vi "Append.vi"(8 "error in":errorcluster, 10 "Digital Waveform in":digitalwaveform(waveform)={"t0"=timestamp(0 s since 1904-01-01), "dt"=1.0, "Y"={"transitions"=[], "data"=[]}}, 11 "Digital Waveform Chart in":refnum<class "Digital Waveform Chart.lvclass">) -> (0 "error out":errorcluster, 2 "Digital Waveform out":digitalwaveform(waveform)={"t0"=timestamp(0 s since 1904-01-01), "dt"=1.0, "Y"={"transitions"=[], "data"=[]}}, 3 "Digital Waveform Chart out":refnum<class "Digital Waveform Chart.lvclass">)   [LabVIEW 2024, in "Digital Waveform Chart.lvclass"]
uses:
  Digital Waveform Chart.lvclass
  Digital Waveform Chart.lvclass/Digital Waveform Chart.ctl
  <vilib>/Waveform/DWDTOps.llb/DWDT Digital Size.vi
  <vilib>/Waveform/DWDTOps.llb/Digital Pattern Generator (Single Value).vi
  <vilib>/Waveform/DWDTOps.llb/DWDT Append Digital Samples.vi
  <vilib>/Waveform/DWDTOps.llb/DWDT Get Waveform Subset.vi
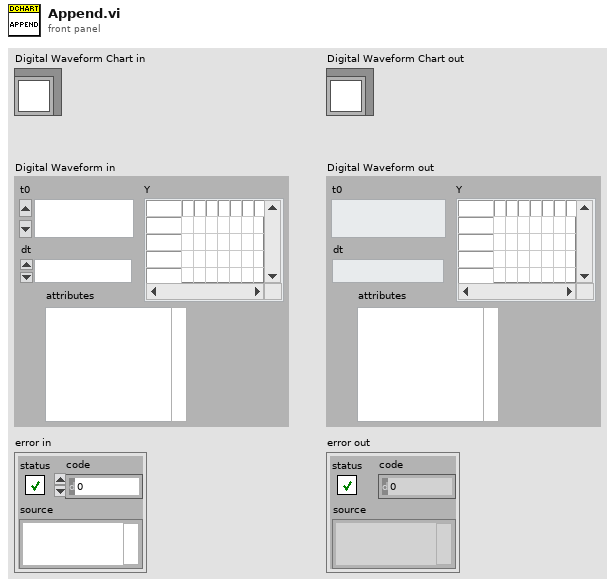
[diagram p1: front panel]
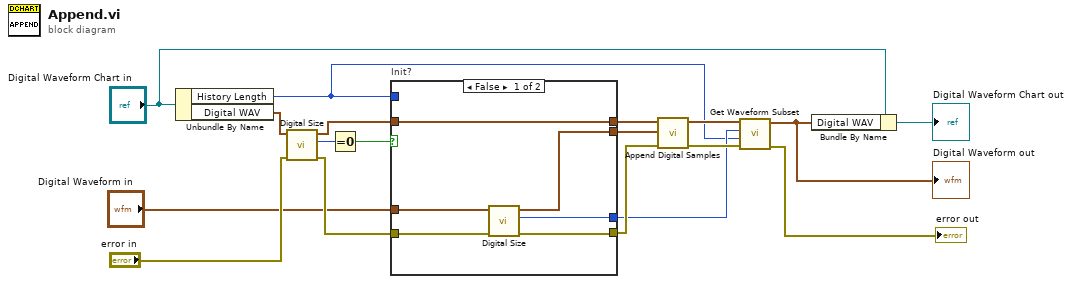
[diagram p0: block diagram]
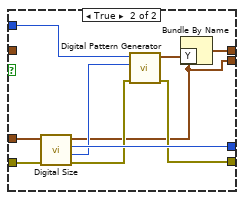
[diagram p2: hidden frame]
diagram:
  n1 = Unbundle By Name("Digital Waveform Chart in") -> ("History Length"=w1:i32, "Digital WAV"=w15:digitalwaveform)
  n2 = call-poly <vilib>:"Digital Size.vi"("error in (no error)"="error in", "digital waveform in"=w15) -> ("error out"=w6:errorcluster, "number of samples"=w16:i32, "digital waveform out"=w9:digitalwaveform)  [unwired: 6 in, 1 out]
  n3 = Equal To 0?(x=w16) -> (x = 0?=w10:bool)
  n4 = case "Init?" shown="False" w10 {
    tunnel: w9 -> [w24 _]
    tunnel: [w24 w33] -> w8
    tunnel: w1 -> [_ w34]
    tunnel: w6 -> [w23 w31]
    tunnel: "Digital Waveform in" -> [w21 w30]
    tunnel: [w22 w26] -> w4
    tunnel: [w19 w29] -> w3
    tunnel: [w20 w25] -> w2
    frame False {
      n5 = call-poly <vilib>:"Digital Size.vi"("error in (no error)"=w23, "digital waveform in"=w21) -> ("error out"=w22:errorcluster, "number of samples"=w19:i32, "digital waveform out"=w20:digitalwaveform)  [unwired: 6 in, 1 out]
    }
    frame True {
      n6 = call-poly <vilib>:"Digital Size.vi"("error in (no error)"=w31, "digital waveform in"=w30) -> ("error out"=w27:errorcluster, "number of signals"=w28:i32, "number of samples"=w29:i32, "digital waveform out"=w25:digitalwaveform)  [unwired: 6 in]
      n7 = call-poly <vilib>:"Digital Pattern Generator.vi"("error in (no error)"=w27, "number of signals"=w28, "number of samples"=w34) -> ("error out"=w26:errorcluster, "digital waveform"=w32:digitalwaveform)  [unwired: 7 in]
      n8 = Bundle By Name(cluster=w25, "Y"=w32) -> (w33:digitalwaveform)
    }
  }
  n9 = call-poly <vilib>:"Append Digital Samples.vi"("error in (no error)"=w4, "digital waveform B"=w2, "digital waveform A"=w8) -> ("error out"=w12:errorcluster, "digital waveform out"=w11:digitalwaveform)  [unwired: 7 in]
  n10 = call-poly <vilib>:"Get Waveform Subset.vi"("error in (no error)"=w12, "duration"=w1, "start samples/time"=w3, "waveform in"=w11) -> ("error out"=→"error out":errorcluster, "waveform out"=w13:digitalwaveform)  [unwired: 2 in, 2 out]
  "Digital Waveform out" <- w13
  n11 = Bundle By Name(cluster="Digital Waveform Chart in", "Digital WAV"=w13) -> (→"Digital Waveform Chart out":refnum<class "Digital Waveform Chart.lvclass">)
